vi "DI9375.vi"() -> ()   [LabVIEW 2023]
uses:
  <vilib>/rvi/interface/nirviOpenFPGA/nirviOpenFPGA.xnode
  <vilib>/rvi/interface/nirviMethod/nirviMethod.xnode
  <vilib>/FPGAPlugInAG/Dynamic/niLvFpga_Run_Dynamic.vi
  <vilib>/rvi/interface/nirviReadWriteControl/nirviReadWriteControl.xnode
  <vilib>/rvi/interface/Simulation/niFpgaSimulationCallBeginRW.vi
  <vilib>/rvi/errors/niLvFpgaAdjustHostInterfaceError.vi
  <vilib>/rvi/interface/nirviCloseFPGA/nirviCloseFPGA.xnode
  <vilib>/FPGAPlugInAG/Dynamic/niLvFpga_Close_Dynamic.vi
  <vilib>/userDefined/High Color/nirio_resource_hc.ctl
panel:
  out "error out":errorcluster
  out "DI 7:0":bool[](array[boolean])
  out "DI 15:8":bool[](array[boolean])
  in  "DO 7:0":bool[](array[boolean])=[FALSE, FALSE, FALSE, FALSE, FALSE, FALSE, FALSE, FALSE]
  in  "DO 15:8":bool[](array[boolean])=[FALSE, FALSE, FALSE, FALSE, FALSE, FALSE, FALSE, FALSE]
  in  "stop":bool
  in  "resource name":T1="RIO0" caption="RIO Device"
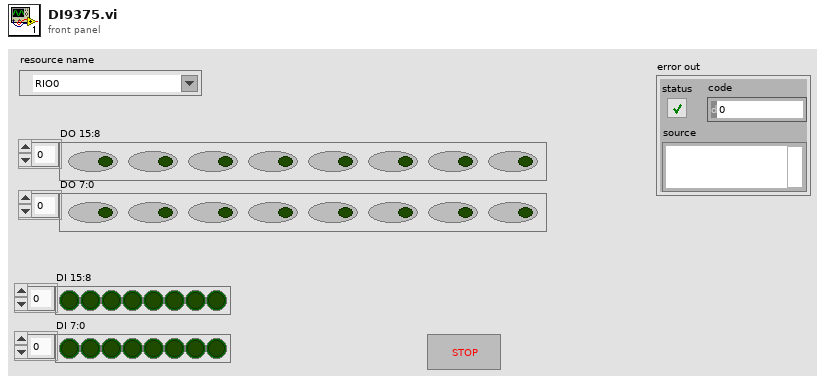
[diagram p1: front panel]
types:
  T1 = typedef "nirio_resource_hc.ctl" = tag
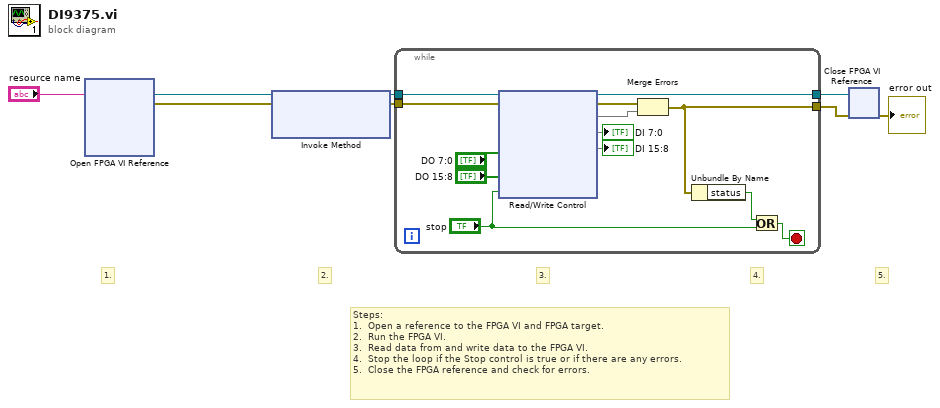
[diagram p0: block diagram]
diagram:
  # "4."
  # "3."
  # "5."
  # "1."
  # "2."
  # "Steps: \n1.  Open a reference to the FPGA VI and FPGA target.\n2.  Run the FPGA VI.\n3.  Read data from and write data to the FPGA VI.\n4.  Stop the loop if the Stop control is true or if there are any errors.\n5.  Close the FPGA reference and check for errors."
  n1 = xnode "Open FPGA VI Reference"("resource name"="resource name") -> ("FPGA VI Reference Out"=w7:refnum<k20>, "error out"=w6:errorcluster)  [unwired: 1 in]
  n2 = xnode "Invoke Method"("FPGA VI Reference In"=w7, "error in"=w6) -> ("FPGA VI Reference Out"=w5:refnum<k20>, "error out"=w4:errorcluster)  [unwired: 1 in]
  n3 = while {
    tunnel: w5 -> [w19]
    tunnel: w4 -> [w18]
    tunnel: [w17] -> w3
    tunnel: [w15] -> w2
    stop <- w20 stop-if-true
    n4 = xnode "Read/Write Control"("FPGA VI Reference In"=w19, "error in"=w18, "DO 7:0"="DO 7:0", "DO 15:8"="DO 15:8", "stop"="stop") -> ("FPGA VI Reference Out"=w17:refnum<k20>, "error out"=w16:errorcluster, "FPGA Error Out"=w14, "DI 7:0"=→"DI 7:0", "DI 15:8"=→"DI 15:8")
    n5 = Merge Errors(w16, w14) -> (w15:errorcluster)
    n6 = Unbundle By Name(w15) -> ("status"=w21:bool)
    n7 = Or(x=w21, y="stop") -> (x .or. y?=w20:bool)
  }
  n8 = xnode "Close FPGA VI Reference"("FPGA VI Reference In"=w3, "error in"=w2) -> ("error out"=→"error out":errorcluster)
